vi "Find square (SubVI).vi"(8 "error in (no error)":errorcluster, 11 "Refnum in":T2) -> (0 "error out":errorcluster, 1 "Calibrated Matches (Geometric Matching 1)":T1[](array[typedef]) {"Correlation Score" format="%.2f"; "Target Template Curve Score" format="%.2f"; "Template Target Curve Score" format="%.2f"; "Bounding Box"."y" format="%.2f"; "Bounding Box"."x" format="%.2f"; "Position"."y" format="%.2f"; "Position"."x" format="%.2f"; "Score" format="%.2f"; "Scale" format="%.2f"; "Angle" format="%.2f"; "Occlusion %" format="%.2f"}, 2 "Number of Matches (Geometric Matching 1) 2":i32, 3 "Refnum out":T2, 5 "Number of Matches (Geometric Matching 1)":i32)   [LabVIEW 2017]
uses:
  <vilib>/vision/Image Controls.llb/IMAQ Image.ctl
  <vilib>/vision/Pattern Matching.llb/IMAQ GM Match Report.ctl
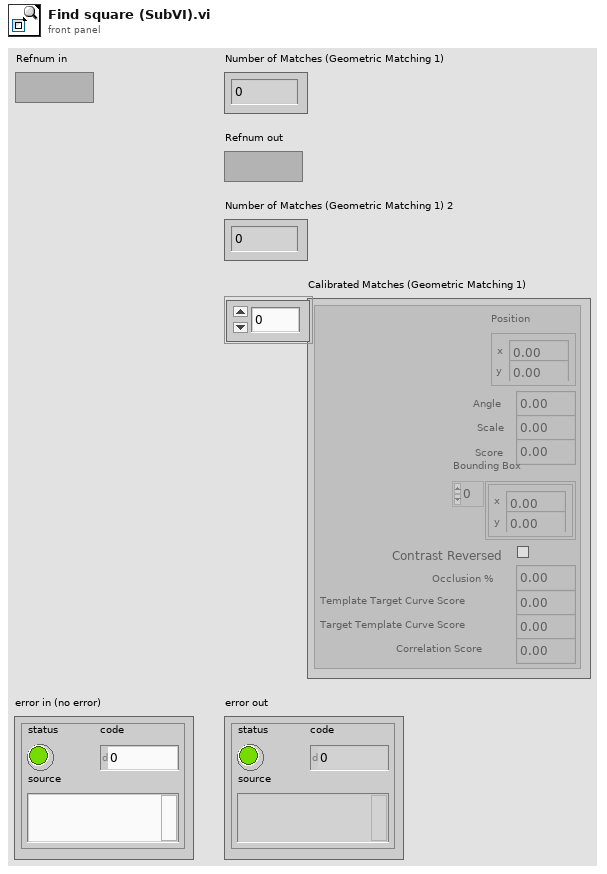
[diagram p1: front panel]
types:
  T1 = typedef "IMAQ GM Match Report.ctl" = cluster{"Position":cluster{"x":sgl, "y":sgl}, "Angle":sgl, "Scale":sgl, "Score":sgl, "Bounding Box":cluster{"x":sgl, "y":sgl}[], "Contrast Reversed":bool, "Occlusion %":sgl, "Template Target Curve Score":sgl, "Target Template Curve Score":sgl, "Correlation Score":sgl}
  T2 = typedef "IMAQ Image.ctl" = refnum<image>
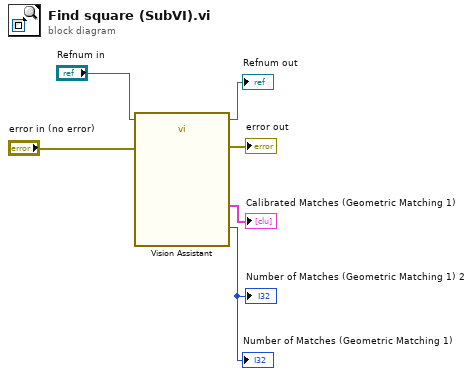
[diagram p0: block diagram]
diagram:
  n1 = call "Vision Assistant"("Image In"="Refnum in", "error in"="error in (no error)") -> ("Image Out"=→"Refnum out":T2, "Calibrated Matches (Geometric Matching 1)"=→"Calibrated Matches (Geometric Matching 1)":T1[], "Number of Matches (Geometric Matching 1)"=→"Number of Matches (Geometric Matching 1)" →"Number of Matches (Geometric Matching 1) 2":i32, "error out"=→"error out":errorcluster)  [unwired: 22 in]
